vi "Example Start Program.vi"() -> ()   [LabVIEW 2010]
uses:
  C:/tf/play/labview/Tinkerforge.dll
  Tinkerforge.dll
panel:
  out "result":string
  in  "program identifier":string="foobar"
  in  "uid":string="XXYYZZ"
  in  "port":i32=4223
  in  "host":string="localhost"
  # "FIXME: Limited to 63 characters"
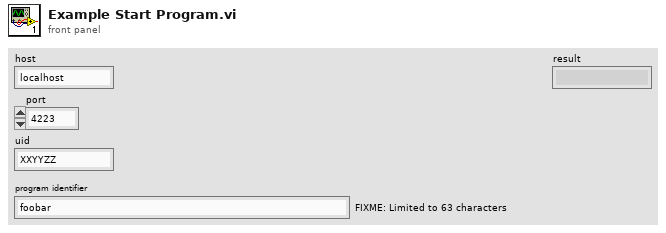
[diagram p1: front panel]
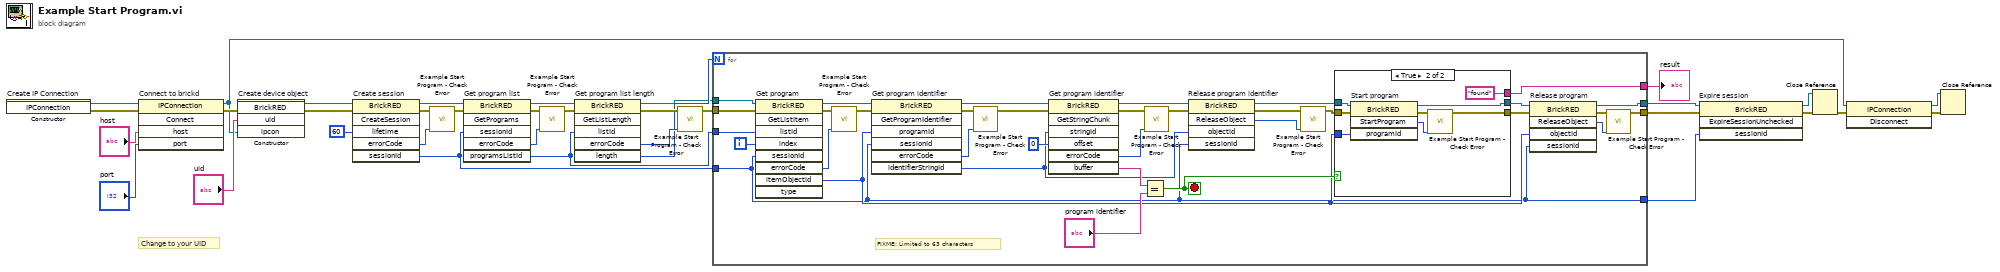
[diagram p0: block diagram]
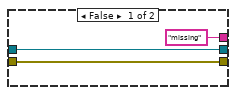
[diagram p2: hidden frame]
diagram:
  # "Change to your UID"
  n1 = constructor on="Create IP Connection" class="IPConnection"() -> (reference out=w34:refnum<k24>, error out=w23:errorcluster)  [unwired: 3 in, 1 out]
  n2 = invoke on="Connect to brickd" class="IPConnection" method="Connect"(reference=w34, error in=w23, "host"="host", "port"="port") -> (reference out=w25:refnum<k24>, error out=w30:errorcluster)  [unwired: 1 in, 3 out]
  n3 = constructor on="Create device object" class="BrickRED"(error in=w30, "uid"="uid", "ipcon"=w25) -> (reference out=w28:refnum<k24>, error out=w29:errorcluster)  [unwired: 2 in, 3 out]
  n4 = invoke on="Create session" class="BrickRED" method="CreateSession"(reference=w28, error in=w29, "lifetime"=i64 60) -> (reference out=w16:refnum<k24>, error out=w21:errorcluster, "errorCode"=w20:u8, "sessionId"=w5:i32)  [unwired: 3 in, 2 out]
  n5 = call "Example Start Program - Check Error.vi"("error code"=w20, "error in"=w21) -> ("error out"=w17:errorcluster)  [unwired: 9 in]
  n6 = invoke on="Get program list" class="BrickRED" method="GetPrograms"(reference=w16, error in=w17, "sessionId"=w5) -> (reference out=w12:refnum<k24>, error out=w15:errorcluster, "errorCode"=w14:u8, "programsListId"=w6:i32)  [unwired: 3 in, 2 out]
  n7 = call "Example Start Program - Check Error.vi"("error code"=w14, "error in"=w15) -> ("error out"=w13:errorcluster)  [unwired: 9 in]
  n8 = invoke on="Get program list length" class="BrickRED" method="GetListLength"(reference=w12, error in=w13, "listId"=w6) -> (reference out=w7:refnum<k24>, error out=w11:errorcluster, "errorCode"=w10:u8, "length"=w9:i32)  [unwired: 3 in, 2 out]
  n9 = call "Example Start Program - Check Error.vi"("error code"=w10, "error in"=w11) -> ("error out"=w8:errorcluster)  [unwired: 9 in]
  n10 = for {
    N: w9 -> [_]
    tunnel: w8 -> [w68]
    tunnel: w7 -> [w67]
    tunnel: w6 -> [w66]
    tunnel: w5 -> [w42]
    tunnel: [w42] -> w4
    tunnel: [w41] -> w3
    tunnel: [w40] -> w2
    tunnel: [w35] -> w1
    i -> [w65]
    stop <- w51 stop-if-true
    # "FIXME: Limited to 63 characters"
    n11 = invoke on="Get program" class="BrickRED" method="GetListItem"(reference=w67, error in=w68, "listId"=w66, "index"=w65, "sessionId"=w42) -> (reference out=w62:refnum<k24>, error out=w64:errorcluster, "errorCode"=w63:u8, "itemObjectId"=w45:i32)  [unwired: 4 in, 5 out]
    n12 = call "Example Start Program - Check Error.vi"("error code"=w63, "error in"=w64) -> ("error out"=w61:errorcluster)  [unwired: 9 in]
    n13 = invoke on="Get program identifier" class="BrickRED" method="GetProgramIdentifier"(reference=w62, error in=w61, "programId"=w45, "sessionId"=w42) -> (reference out=w56:refnum<k24>, error out=w60:errorcluster, "errorCode"=w59:u8, "identifierStringId"=w48:i32)  [unwired: 3 in, 3 out]
    n14 = call "Example Start Program - Check Error.vi"("error code"=w59, "error in"=w60) -> ("error out"=w57:errorcluster)  [unwired: 9 in]
    n15 = invoke on="Get program identifier" class="BrickRED" method="GetStringChunk"(reference=w56, error in=w57, "stringId"=w48, "offset"=i64 0) -> (reference out=w49:refnum<k24>, error out=w55:errorcluster, "errorCode"=w54:u8, "buffer"=w53:string)  [unwired: 3 in, 3 out]
    n16 = Equal?(x=w53, y="program identifier") -> (x = y?=w51:bool)
    n17 = call "Example Start Program - Check Error.vi"("error code"=w54, "error in"=w55) -> ("error out"=w50:errorcluster)  [unwired: 9 in]
    n18 = invoke on="Release program identifier" class="BrickRED" method="ReleaseObject"(reference=w49, error in=w50, "objectId"=w48, "sessionId"=w42) -> (reference out=w36:refnum<k24>, error out=w39:errorcluster, "ReleaseObject"=w37:u8)  [unwired: 1 in, 2 out]
    n19 = call "Example Start Program - Check Error.vi"("error code"=w37, "error in"=w39) -> ("error out"=w38:errorcluster)  [unwired: 9 in]
    n20 = case shown="True" w51 {
      tunnel: w45 -> [_ w79]
      tunnel: w38 -> [w70 w78]
      tunnel: w36 -> [w71 w77]
      tunnel: [w70 w74] -> w47
      tunnel: [w71 w73] -> w46
      tunnel: ["missing" "found"] -> w35
      frame False {
      }
      frame True {
        n21 = invoke on="Start program" class="BrickRED" method="StartProgram"(reference=w77, error in=w78, "programId"=w79) -> (reference out=w73:refnum<k24>, error out=w75:errorcluster, "StartProgram"=w76:u8)  [unwired: 1 in, 1 out]
        n22 = call "Example Start Program - Check Error.vi"("error code"=w76, "error in"=w75) -> ("error out"=w74:errorcluster)  [unwired: 9 in]
      }
    }
    n23 = invoke on="Release program" class="BrickRED" method="ReleaseObject"(reference=w46, error in=w47, "objectId"=w45, "sessionId"=w42) -> (reference out=w40:refnum<k24>, error out=w43:errorcluster, "ReleaseObject"=w44:u8)  [unwired: 1 in, 2 out]
    n24 = call "Example Start Program - Check Error.vi"("error code"=w44, "error in"=w43) -> ("error out"=w41:errorcluster)  [unwired: 9 in]
  }
  "result" <- w1
  n25 = invoke on="Expire session" class="BrickRED" method="ExpireSessionUnchecked"(reference=w2, error in=w3, "sessionId"=w4) -> (reference out=w19:refnum<k24>, error out=w18:errorcluster)  [unwired: 1 in, 2 out]
  n26 = Close Reference(reference=w19, error in (no error)=w18) -> (error out=w27:errorcluster)
  n27 = invoke class="IPConnection" method="Disconnect"(reference=w25, error in=w27) -> (reference out=w24:refnum<k24>, error out=w26:errorcluster)  [unwired: 1 in, 1 out]
  n28 = Close Reference(reference=w24, error in (no error)=w26) -> ()  [unwired: 1 out]
